vi "saveDataNodeEnd.vi"(8 "error in (no error)":errorcluster, 9 "indent":i32, 10 "XML Refnum in":refnum<file>, 11 "xceDataNode in":refnum<class "xceDataNode.lvclass">) -> (0 "error out":errorcluster, 2 "XML Refnum out":refnum<file>, 3 "xceDataNode out":refnum<class "xceDataNode.lvclass">)   [LabVIEW 2013, in "xceDataNode.lvclass"]
doc: "Ends the process of saving a xceData Node to an XML formatted file."
uses:
  xceDataNode.lvclass
  xceNode/xceNode.lvclass
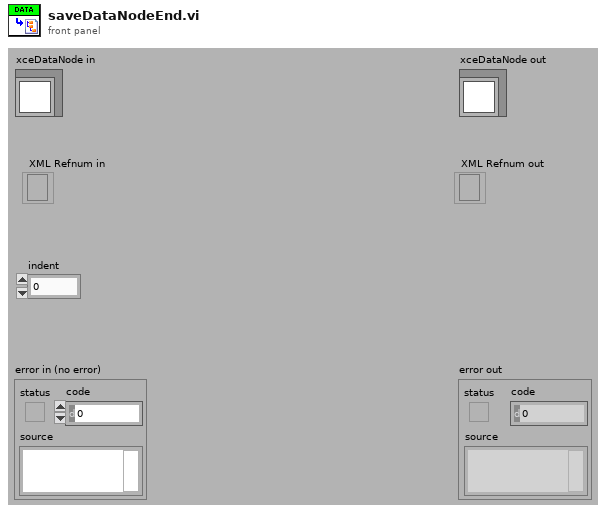
[diagram p1: front panel]
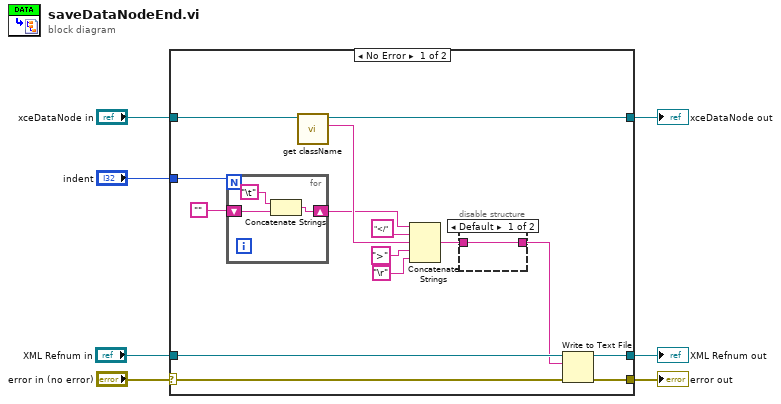
[diagram p0: block diagram]
diagram:
  n1 = case shown="No Error" "error in (no error)" {
    selector: "error in (no error)" -> [w15 w29]
    tunnel: [w8 w29] -> w6
    tunnel: [w10 w28] -> w4
    tunnel: "xceDataNode in" -> [w21 w28]
    tunnel: "indent" -> [w12 _]
    tunnel: "XML Refnum in" -> [w14 w27]
    tunnel: [w9 w27] -> w1
    frame No Error {
      n2 = for {
        N: w12 -> [_]
        shift-right: [w26] -> w11
        shift-left: "" -> [w25]
        n3 = Concatenate Strings("\t", w25) -> (w26:string)
      }
      n4 = call "get className.vi"("xceNode in"=w21) -> ("Class name"=w19:string, "xceNode out"=w10:refnum<class "xceDataNode.lvclass">)  [unwired: 8 in, 1 out]
      n5 = Concatenate Strings(w11, "</", w19, ">", "\r") -> (w16:string)
      n6 = disable-structure shown="Default" {
        disable-tunnel: w16 -> [w23 _]
        disable-tunnel: [w23 _] -> w13
        frame condition #0 (active) {
        }
        frame condition #1 {
        }
      }
      n7 = Write to Text File(file (use dialog)=w14, text=w13, error in=w15) -> (refnum out=w9:refnum<file>, error out=w8:errorcluster)  [unwired: 1 in, 1 out]
    }
    frame Error {
    }
  }
  "error out" <- w6
  "xceDataNode out" <- w4
  "XML Refnum out" <- w1
